vi "User menu handler.vi"(9 "UI queue":refnum<queue>, 11 "User Menu ItemTag":string) -> (0 "error out":errorcluster)   [LabVIEW 2020]
uses:
  Queue/Message Queue/Typedefs/Message Cluster.ctl
  Global Variables/General Globals.vi
  Configuration code/Calibration/Globals/gl_Calibration globals.vi
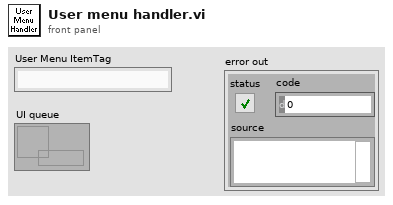
[diagram p1: front panel]
types:
  T1 = enum16{"Software Init", "User menu", "Switch User button"}
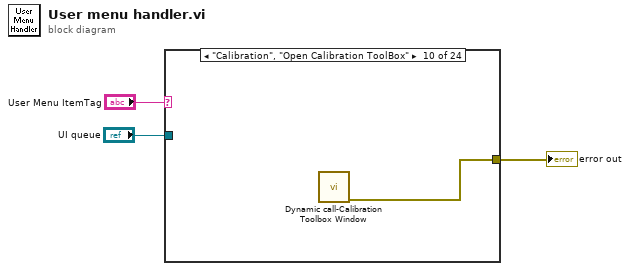
[diagram p0: block diagram]
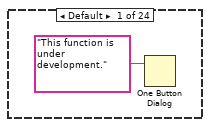
[diagram p2: hidden frame]
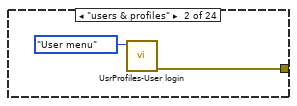
[diagram p3: hidden frame]
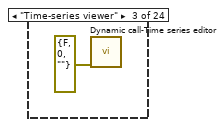
[diagram p4: hidden frame]
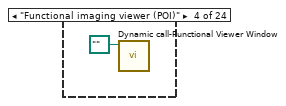
[diagram p5: hidden frame]
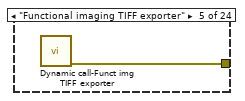
[diagram p6: hidden frame]
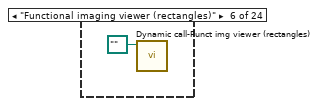
[diagram p7: hidden frame]
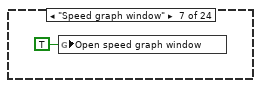
[diagram p8: hidden frame]
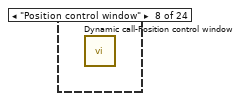
[diagram p9: hidden frame]
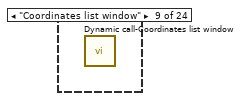
[diagram p10: hidden frame]
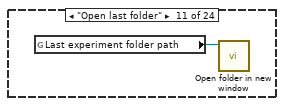
[diagram p11: hidden frame]
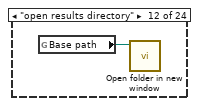
[diagram p12: hidden frame]
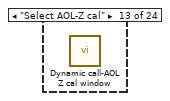
[diagram p13: hidden frame]
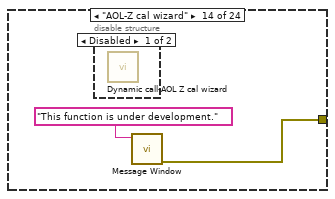
[diagram p14: hidden frame]
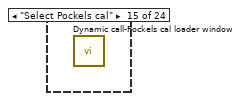
[diagram p16: hidden frame]
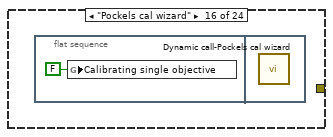
[diagram p17: hidden frame]
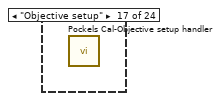
[diagram p18: hidden frame]
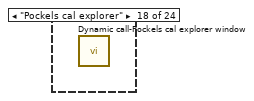
[diagram p19: hidden frame]
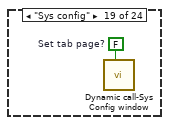
[diagram p20: hidden frame]
diagram:
  n1 = case shown="\"Calibration\", \"Open Calibration ToolBox\"" "User Menu ItemTag" {
    tunnel: "UI queue" -> [_ _ _ _ _ _ _ _ _ _ _ _ _ _ _ _ _ _ _ _ _ _ w21 w23]
    tunnel: [_ w6 _ _ w9 _ _ _ _ w12 _ _ _ w15 _ _ _ _ _ _ _ _ w20 w22] -> w1
    frame Default {
      n2 = One Button Dialog(message="This function is under development.") -> ()  [unwired: 1 in, 1 out]
    }
    frame "users & profiles" {
      n3 = call "UsrProfiles-User login.vi"("Access source (Soft init)"=T1."User menu") -> ("error out"=w6:errorcluster)  [unwired: 10 in]
    }
    frame "Time-series viewer" {
      n4 = call "Dynamic call-Time series editor.vi"("error in (no error)"=errorcluster {"status"=FALSE, "code"=0, "source"=""}) -> ()  [unwired: 10 in, 1 out]
    }
    frame "Functional imaging viewer (POI)" {
      n5 = call "Dynamic call-Functional Viewer Window.vi"("Experiment data folder path"=path "") -> ()  [unwired: 11 in]
    }
    frame "Functional imaging TIFF exporter" {
      n6 = call "Dynamic call-Funct img TIFF exporter.vi"() -> ("error out"=w9:errorcluster)  [unwired: 11 in]
    }
    frame "Functional imaging viewer (rectangles)" {
      n7 = call "Dynamic call-Funct img viewer (rectangles).vi"("Experiment Path"=path "") -> ()  [unwired: 10 in, 1 out]
    }
    frame "Speed graph window" {
      n8 = global write "General Globals.vi" "Open speed graph window"(TRUE ("Open speed graph window")) -> ()
    }
    frame "Position control window" {
      n9 = call "Dynamic call-Position control window.vi"() -> ()  [unwired: 11 in, 1 out]
    }
    frame "Coordinates list window" {
      n10 = call "Dynamic call-Coordinates list window.vi"() -> ()  [unwired: 11 in, 1 out]
    }
    frame "Calibration", "Open Calibration ToolBox" {
      n11 = call "Dynamic call-Calibration Toolbox Window.vi"() -> ("error out"=w12:errorcluster)  [unwired: 11 in]
    }
    frame "Open last folder" {
      n12 = global read "General Globals.vi" "Last experiment folder path"() -> (w13:path)
      n13 = call "Open folder in new window.vi"("Directory to open"=w13) -> ()  [unwired: 10 in, 1 out]
    }
    frame "open results directory" {
      n14 = global read "General Globals.vi" "Base path"() -> (w14:path)
      n15 = call "Open folder in new window.vi"("Directory to open"=w14) -> ()  [unwired: 10 in, 1 out]
    }
    frame "Select AOL-Z cal" {
      n16 = call "Dynamic call-AOL Z cal window.vi"() -> ()  [unwired: 11 in, 1 out]
    }
    frame "AOL-Z cal wizard" {
      n17 = disable-structure shown="Disabled" {
        frame Disabled {
          n18 = call "Dynamic call-AOL Z cal wizard.vi"() -> ()  [unwired: 11 in, 1 out]
        }
        frame Enabled {
        }
      }
      n19 = call "Message Window.vi"("Message string"="This function is under development.") -> ("error out (no error)"=w15:errorcluster)  [unwired: 10 in]
    }
    frame "Select Pockels cal" {
      n20 = call "Dynamic call-Pockels cal loader window.vi"() -> ()  [unwired: 11 in, 1 out]
    }
    frame "Pockels cal wizard" {
      n21 = flat-sequence {
        frame #0 {
          n22 = global write "gl_Calibration globals.vi" "Calibrating single objective"(FALSE ("Calibrating single objective")) -> ()
        }
        frame #1 {
          n23 = call "Dynamic call-Pockels cal wizard.vi"() -> ()  [unwired: 11 in, 1 out]
        }
      }
    }
    frame "Objective setup" {
      n24 = call "Pockels Cal-Objective setup handler.vi"() -> ()  [unwired: 12 in]
    }
    frame "Pockels cal explorer" {
      n25 = call "Dynamic call-Pockels cal explorer window.vi"() -> ()  [unwired: 11 in, 1 out]
    }
    frame "Sys config" {
      w18 = FALSE  # Set tab page?
      n26 = call "Dynamic call-Sys Config window.vi"("Set tab page? (F)"=w18) -> ()  [unwired: 10 in, 1 out]
    }
    frame "Help" {
      n27 = Control Help Window(1:TRUE ("Show")) -> ()  [unwired: 1 in]
    }
    frame "Web" {
      n28 = call "SilverLab Web.vi"() -> ()  [unwired: 12 in]
    }
    frame "About" {
      n29 = call "Window-About.vi"() -> ()  [unwired: 12 in]
    }
    frame "shut down" {
      n30 = disable-structure shown="Disabled" {
        frame Disabled {
          n31 = call "Window-Exit window.vi"() -> ()  [unwired: 10 in, 2 out]
        }
        frame Enabled {
        }
      }
      n32 = call "Event handler-Exit.vi"("UI queue"=w21) -> ("error out"=w20:errorcluster)  [unwired: 9 in, 1 out]
    }
    frame "restart" {
      n33 = disable-structure shown="Disabled" {
        frame Disabled {
          n34 = call "Window-Restart window.vi"() -> ()  [unwired: 10 in, 2 out]
        }
        frame Enabled {
        }
      }
      n35 = call "Event handler-Restart.vi"("Queue in"=w23) -> ("error out"=w22:errorcluster)  [unwired: 10 in]
    }
  }
  "error out" <- w1
